vi "e.gate HighSpeedPort Read Buffer - CORE.vi"(2 "Backtime":dbl, 3 "Iteration":i32=1000, 4 "force Backtime":bool, 5 "No Erasing":bool, 7 "error in (no error)":errorcluster, 8 "Configuration in":T1) -> (18 "Configuration out":T1, 21 "data array (binary)":u8[](array[numeric]), 24 "StructureID":i32, 27 "error out":errorcluster)   [LabVIEW 2016]
doc: "This VI is used to receive binary buffer data from controller and decode the state information's at the beginning."
uses:
  e.gate Configuration.ctl
  e.gate Channel Data.ctl
  e.gate Data Type.ctl
  e.gate Protocol Type.ctl
  e.gate Module  Data.ctl
  e.gateHSP_DLLhandle.ctl
panel:
  out "data out":string
  out "LastTransferState":i32
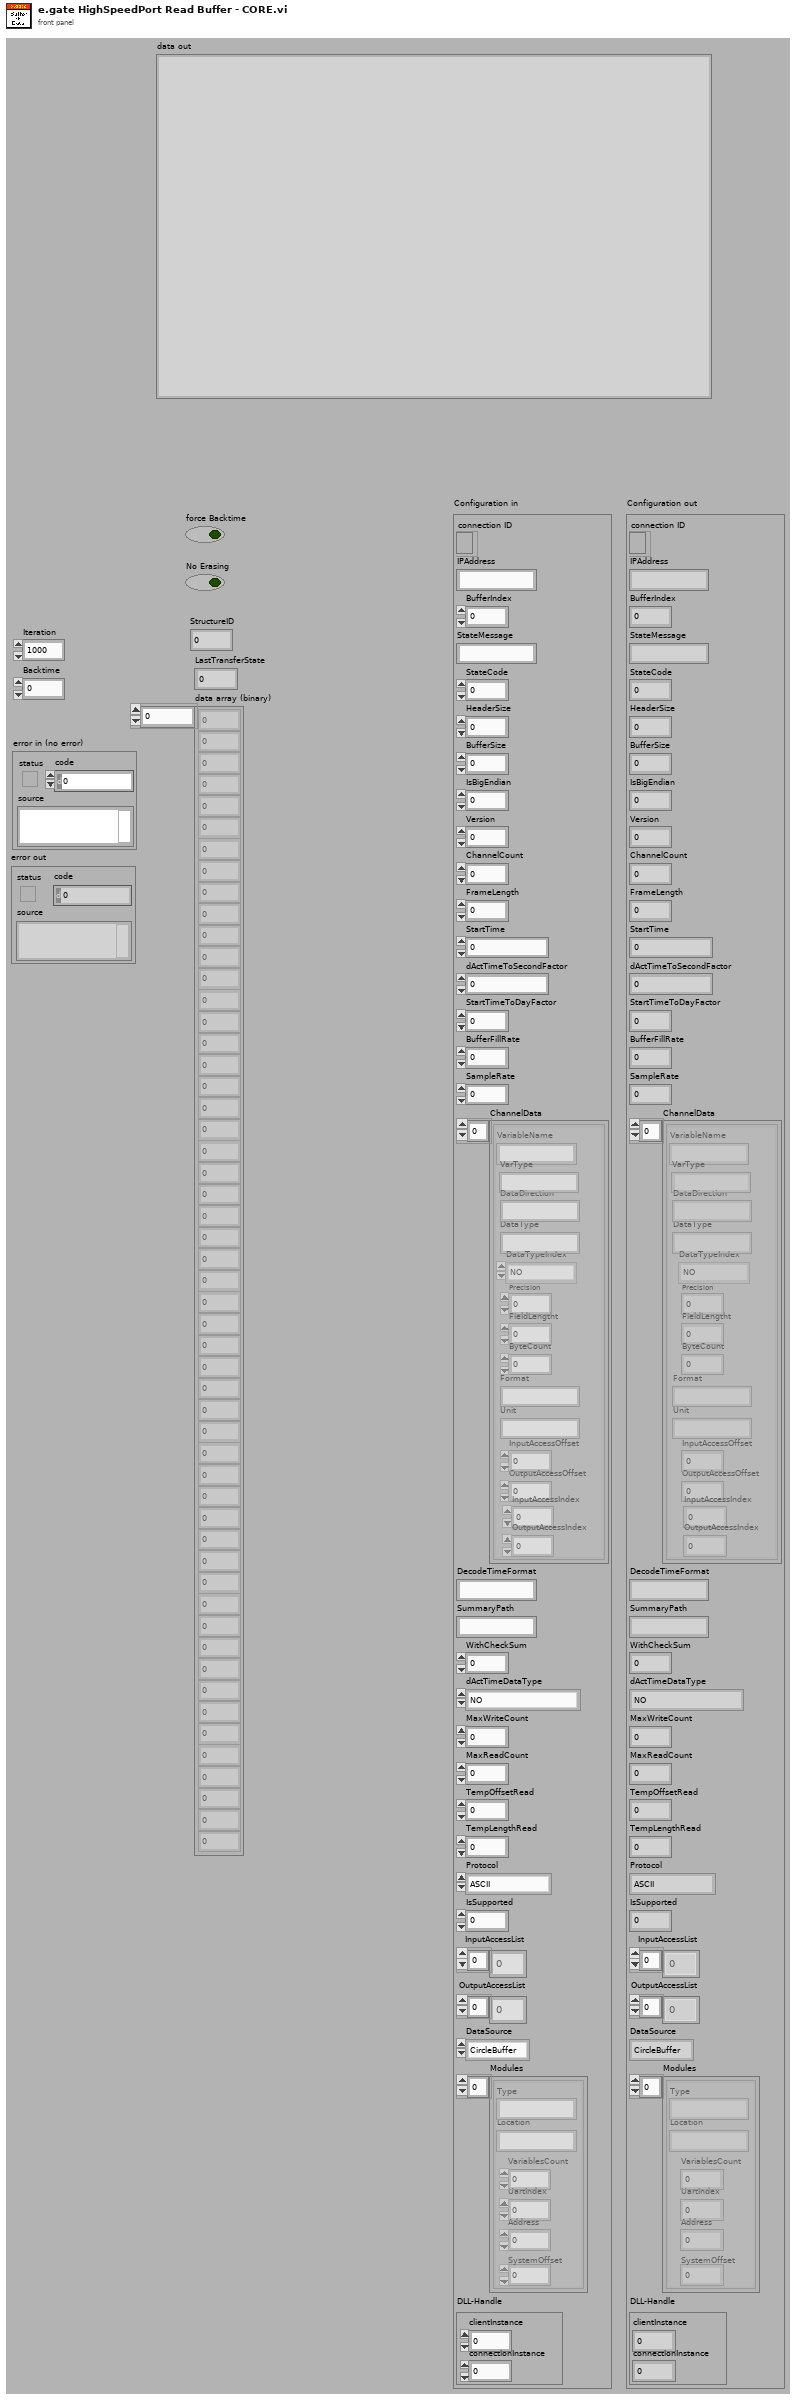
[diagram p1: front panel]
types:
  T1 = typedef "e.gate Configuration.ctl" = cluster{"connection ID":refnum<k5>, "IPAddress":string, "BufferIndex":i32, "StateMessage":string, "StateCode":i8, "HeaderSize":i32, "BufferSize":i32, "IsBigEndian":i32, "Version":i32, "ChannelCount":i32, "FrameLength":i32, "StartTime":dbl, "dActTimeToSecondFactor":dbl, "StartTimeToDayFactor":dbl, "BufferFillRate":dbl, "SampleRate":dbl, "ChannelData":T2[], "DecodeTimeFormat":string, "SummaryPath":string, "WithCheckSum":i32, "dActTimeDataType":T3, "MaxWriteCount":i32, "MaxReadCount":i32, "TempOffsetRead":i32, "TempLengthRead":i32, "Protocol":T4, "IsSupported":i32, "InputAccessList":i32[], "OutputAccessList":i32[], "DataSource":enum16{"CircleBuffer", "test.con Logger", "test.con Archive"}, "Modules":T5[], "DLL-Handle":T6}
  T2 = typedef "e.gate Channel Data.ctl" = cluster{"VariableName":string, "DataDirection":string, "DataType":string, "DataTypeIndex":T3, "Precision":i16, "FieldLengtht":i16, "ByteCount":i32, "Format":string, "Unit":string, "InputAccessOffset":i32, "OutputAccessOffset":i16, "InputAccessIndex":i16, "OutputAccessIndex":i16, "VarType":string}
  T3 = typedef "e.gate Data Type.ctl" = enum16{"NO", "BOOL", "SINT8", "USINT8", "SINT16", "USINT16", "SINT32", "USINT32", "FLOAT", "SET8", "SET16", "SET32", "DOUBLE", "SINT64", "USINT64", "SET64"}
  T4 = typedef "e.gate Protocol Type.ctl" = enum16{"ASCII", "HighspeedPort Online", "HighspeedPort Buffer", "eGateHighspeedPortDLL "}
  T5 = typedef "e.gate Module  Data.ctl" = cluster{"Type":string, "Location":string, "VariablesCount":i16, "UartIndex":i16, "Address":i16, "SystemOffset":i16}
  T6 = typedef "e.gateHSP_DLLhandle.ctl" = cluster{"clientInstance":i32, "connectionInstance":i32}
  T7 = enum16{"Standard", "Buffered", "CRLF", "Immediate"}
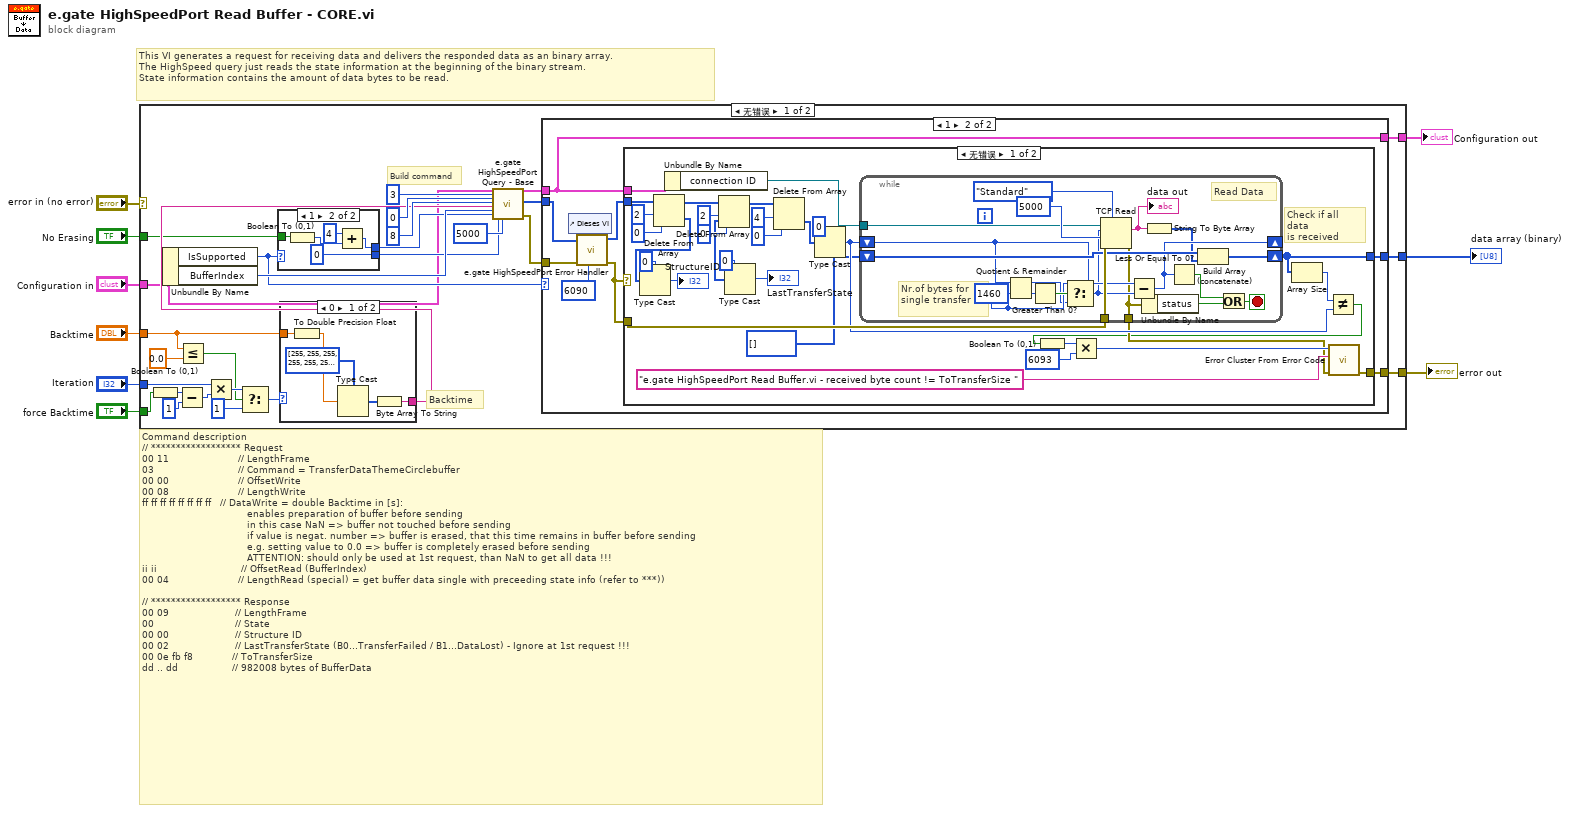
[diagram p0: block diagram]
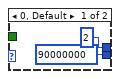
[diagram p2: hidden frame]
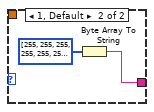
[diagram p5: hidden frame]
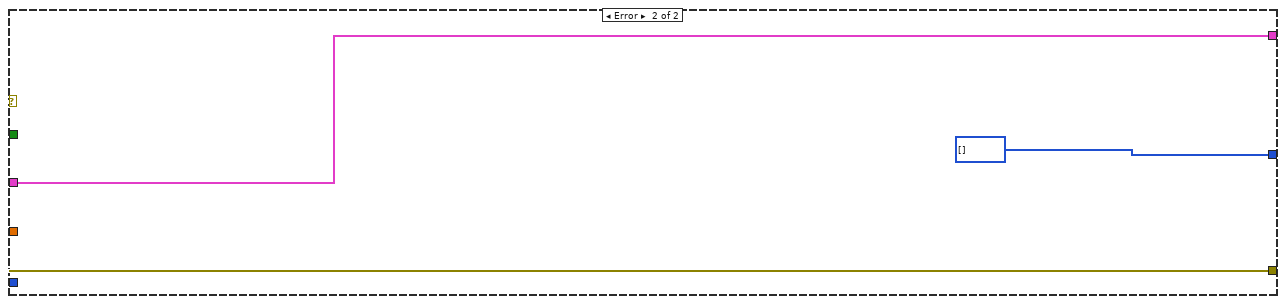
[diagram p6: hidden frame]
diagram:
  # "Command description\n// ****************** Request\n00 11\t\t\t\t\t                 \t// LengthFrame\n03\t\t\t\t\t\t                     \t// Command = TransferDataThemeCirclebuffer\n00 00\t\t\t\t\t                 \t// OffsetWrite\n00 08\t\t\t\t                 \t\t// LengthWrite\nff ff ff ff ff ff ff ff\t\t // DataWrite = double Backtime in [s]:\n\t\t\t\t\t\t\t                            enables preparation of buffer before sending\n\t\t\t\t\t\t\t                           \tin this case NaN => buffer not touched before sending\n\t\t\t\t\t\t                           \t\tif value is negat. number => buffer is erased, that this time remains in buffer before sending\n\t\t\t\t\t\t                           \t\te.g. setting value to 0.0 => buffer is completely erased before sending\n\t\t\t\t\t\t\t                           \tATTENTION: should only be used at 1st request, than NaN to get all data !!!\nii ii\t\t\t\t\t\t                      // OffsetRead (BufferIndex)\n00 04\t\t\t\t\t                 \t// LengthRead (special) = get buffer data single with preceeding state info (refer to ***))\n\n// ****************** Response\n00 09\t\t\t\t\t                \t// LengthFrame\n00\t\t\t\t\t                    \t\t// State\n00 00\t\t\t\t\t                \t// Structure ID\n00 02\t\t\t\t\t                \t// LastTransferState (B0...TransferFailed / B1...DataLost) - Ignore at 1st request !!!\n00 0e fb f8\t\t\t          // ToTransferSize\ndd .. dd\t\t\t             \t\t// 982008 bytes of BufferData"
  # "This VI generates a request for receiving data and delivers the responded data as an binary array.\nThe HighSpeed query just reads the state information at the beginning of the binary stream. \nState information contains the amount of data bytes to be read."
  n1 = case shown="无错误" "error in (no error)" {
    selector: "error in (no error)" -> [_ w118]
    tunnel: "Backtime" -> [w18 _]
    tunnel: [w37 u8[] [] ("unsigned byte array")] -> w8
    tunnel: [w36 w118] -> w5
    tunnel: "Configuration in" -> [w12 w116]
    tunnel: "Iteration" -> [w25 _]
    tunnel: "force Backtime" -> [w21 _]
    tunnel: "No Erasing" -> [w20 _]
    tunnel: [w11 w116] -> w1
    frame No Error {
      # "Backtime"
      # "Build command"
      n2 = Boolean To (0,1)(Boolean=w21) -> (0, 1=w22:i16)
      n3 = Unbundle By Name(w12) -> ("IsSupported"=w19:i32, "BufferIndex"=w29:i32)
      n4 = Subtract(x=w22, y=1) -> (x-y=w24:i32)
      n5 = Less Or Equal?(x=w18, y=0.0) -> (x <= y?=w14:bool)
      n6 = Multiply(x=w25, y=w24) -> (x*y=w16:i32)
      n7 = Select(t=w16, s=w14, f=1) -> (s? t:f=w15:i32)
      n8 = case shown="1" w19 {
        tunnel: [90000000 ("LengthRead") 0 ("LengthRead")] -> w27
        tunnel: [2 ("LengthRead") w43] -> w26
        tunnel: w20 -> [_ w40]
        frame 0, Default {
        }
        frame 1 {
          n9 = Boolean To (0,1)(Boolean=w40) -> (0, 1=w41:i16)
          n10 = Add(x=4 ("LengthRead"), y=w41) -> (x+y=w43:i32)
        }
      }
      n11 = case shown="0" w15 {
        tunnel: [w109 w115] -> w28
        tunnel: w18 -> [w113 _]
        frame 0 {
          n12 = To Double Precision Float(number=w113) -> (double precision float=w111:dbl)
          n13 = Type Cast(type=u8[] [255, 255, 255, 255, 255, 255, 255, 255] ("Vorzeichenloses Byte-Array"), x=w111) -> (*(type *) &x=w112:u8[])
          n14 = Byte Array To String(unsigned byte array=w112) -> (string=w109:string)
        }
        frame 1, Default {
          n15 = Byte Array To String(unsigned byte array=u8[] [255, 255, 255, 255, 255, 255, 255, 255] ("Vorzeichenloses Byte-Array")) -> (string=w115:string)
        }
      }
      n16 = call "e.gate HighSpeedPort Query - Base.vi"("e.gate Configuration in"=w12, "Command"=3, "OffsetWrite"=0, "LengthWrite"=8, "DataWrite"=w28, "OffsetRead"=w29, "LengthRead"=w26, "TCP LengthReadt"=w27, "Timeout (1000)"=5000) -> ("e.gate Configuration out"=w30:T1, "Data (out binary)"=w31:u8[], "error out"=w10:errorcluster)  [unwired: 1 in, 15 out]
      n17 = case shown="1" w19 {
        tunnel: [w47 w56] -> w37
        tunnel: [w45 w55] -> w36
        tunnel: w31 -> [w47 w51]
        tunnel: w30 -> [w46 w54]
        tunnel: [w46 w54] -> w11
        tunnel: w10 -> [w45 w50]
        frame 0, Default {
        }
        frame 1 {
          n18 = control-ref of="Dieses VI"() -> (w53:refnum<vi>)
          n19 = call "e.gate HighSpeedPort Error Handler.vi"("error code start index"=6090, "VI reference"=w53, "error in (no error)"=w50, "binary data in"=w51) -> ("error out"=w48:errorcluster, "binary out"=w49:u8[])  [unwired: 6 out]
          n20 = case shown="无错误" w48 {
            tunnel: [w59 w107] -> w56
            tunnel: [w87 w108] -> w55
            tunnel: w54 -> [w86 _]
            tunnel: w49 -> [w85 w107]
            tunnel: w48 -> [w84 w108]
            frame No Error {
              # "Check if all data \nis received"
              n21 = Delete From Array(array=w85, length=2 ("Länge"), index=0 ("Index")) -> (deleted portion=w73:u8[], array with subset deleted=w81:u8[])
              n22 = Type Cast(type=i16 0, x=w73) -> (*(type *) &x=→"StructureID":i16)
              n23 = Unbundle By Name(w86) -> ("connection ID"=w60:refnum<k5>)
              n24 = Delete From Array(array=w81, length=2 ("Länge"), index=0 ("Index")) -> (deleted portion=w72:u8[], array with subset deleted=w76:u8[])
              n25 = Type Cast(type=i16 0, x=w72) -> (*(type *) &x=→"LastTransferState":i16)
              n26 = Delete From Array(array=w76, length=4 ("Länge"), index=0 ("Index")) -> (deleted portion=w70:u8[])  [unwired: 1 out]
              n27 = Type Cast(type=0, x=w70) -> (*(type *) &x=w68:i32)
              n28 = while {
                tunnel: w84 -> [w106]
                tunnel: [w93] -> w61
                tunnel: w60 -> [w102]
                shift-right: [w100] -> w59
                shift-left: u8[] [] ("unsigned byte array") -> [w101]
                shift-right: [w91] -> _
                shift-left: w68 -> [w95]
                stop <- w92 stop-if-true
                w97 = 1460 ("y")
                # "Nr.of bytes for\nsingle transfer"
                # "Read Data"
                n29 = Quotient & Remainder(x=w95, y=w97) -> (x-y*floor(x/y)=w96:i32, floor(x/y)=w99:i32)
                n30 = Greater Than 0?(x=w99) -> (x > 0?=w98:bool)
                n31 = Select(t=w97, s=w98, f=w96) -> (s? t:f=w94:i32)
                n32 = TCP Read ("TCP: Lesen")(connection ID=w102, bytes to read=w94, error in (no error)=w106, 7:T7."Standard" ("Modus (Standard)"), 9:5000 ("Timeout in ms (25000)")) -> (data out=w105:string, error out=w93:errorcluster)  [unwired: 1 out]
                "data out" <- w105
                n33 = Subtract(x=w95, y=w94) -> (x-y=w91:i32)
                n34 = Unbundle By Name(w93) -> ("status"=w88:bool)
                n35 = String To Byte Array(string=w105) -> (unsigned byte array=w89:u8[])
                n36 = Less Or Equal To 0?(x=w91) -> (x <= 0?=w90:bool)
                n37 = Build Array (concatenate)(w101, w89) -> (w100:u8[])
                n38 = Or(x=w90, y=w88) -> (x .or. y?=w92:bool)
              }
              n39 = Array Size(array=w59) -> (size(s)=w69:i32)
              n40 = Not Equal?(x=w69, y=w68) -> (x != y?=w57:bool)
              n41 = Boolean To (0,1)(Boolean=w57) -> (0, 1=w65:i16)
              n42 = Multiply(x=w65, y=i16 6093) -> (x*y=w64:i16)
              n43 = call <vilib>:"Error Cluster From Error Code.vi"("error in (no error)"=w61, "error message (\"\")"="e.gate HighSpeedPort Read Buffer.vi - received byte count != ToTransferSize " ("error message (\"\")"), "error code (0)"=w64) -> ("error out"=w87:errorcluster)  [unwired: 1 in, 5 out]
            }
            frame Error {
            }
          }
        }
      }
    }
    frame Error {
    }
  }
  "data array (binary)" <- w8
  "Configuration out" <- w1
  "error out" <- w5
